vi "Operate Result.vi"(0 "reference":refnum<k24>, 11 "error in (no error)":errorcluster) -> (15 "error out":errorcluster)   [LabVIEW 2020, in "HslCommunication.lvlib"]
uses:
  HslCommunication.lvlib
  D:/Git/Labview-Libraries/Libraries/HslCommunication/_Dependenciecs/HslCommunication.dll
  _Dependenciecs/HslCommunication.dll
panel:
  in  "LogNetStatistics":refnum<k24>
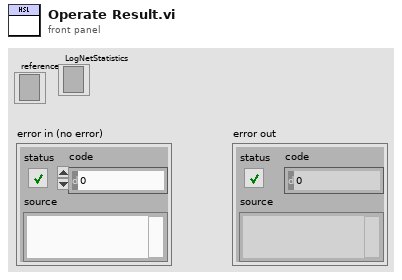
[diagram p1: front panel]
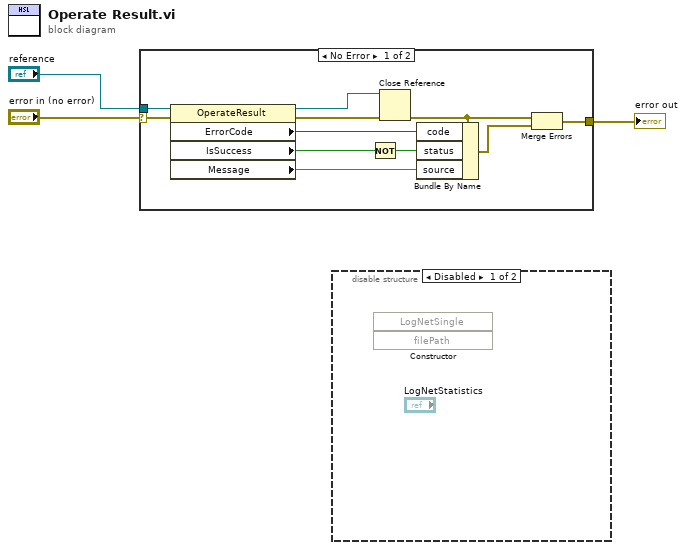
[diagram p0: block diagram]
diagram:
  n1 = case shown="No Error" "error in (no error)" {
    selector: "error in (no error)" -> [w5 w15]
    tunnel: [w6 w15] -> w3
    tunnel: "reference" -> [w4 _]
    frame No Error {
      n2 = property class="OperateResult"(reference=w4, error in=w5) -> (reference out=w9:refnum<k24>, error out=w8:errorcluster, "ErrorCode"=w12:i32, "IsSuccess"=w7:bool, "Message"=w10:string)
      n3 = Not(x=w7) -> (.not. x?=w11:bool)
      n4 = Close Reference(reference=w9, error in (no error)=w8) -> (error out=w13:errorcluster)
      n5 = Bundle By Name(cluster=w13, "code"=w12, "status"=w11, "source"=w10) -> (w14:errorcluster)
      n6 = Merge Errors(w13, w14) -> (w6:errorcluster)
    }
    frame Error {
    }
  }
  "error out" <- w3
  n7 = disable-structure shown="Disabled" {
    frame Disabled {
      n8 = constructor class="LogNetSingle"() -> ()  [unwired: 4 in, 4 out]
    }
    frame Enabled {
    }
  }
